vi "CameraServo.vi"(1 "Y":dbl, 2 "X":dbl) -> ()   [LabVIEW 2014]
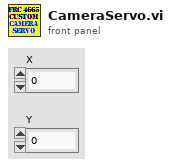
[diagram p1: front panel]
types:
  T1 = typedef "WPI_ServoDeviceRef.ctl" = cluster{"DeviceStatus":errorcluster, "Controller":T2, "PWM Channel":T3, "DeadBand":T4}
  T2 = typedef "FPGA_TypedefDigitalModule.ctl" = enum16{"Controller 1"}
  T3 = typedef "FPGA_DIOPWMChannel.ctl" = enum8{"PWM 0", "PWM 1", "PWM 2", "PWM 3", "PWM 4", "PWM 5", "PWM 6", "PWM 7", "PWM 8", "PWM 9", "PWM MXP 0", "PWM MXP 1", "PWM MXP 2", "PWM MXP 3", "PWM MXP 4", "PWM MXP 5", "PWM MXP 6", "PWM MXP 7", "PWM MXP 8", "PWM MXP 9", "Invalid"}
  T4 = typedef "WPI_PWMDeadband.ctl" = cluster{"Name":string, "maxPositivePwm":i32, "minPositivePwm":i32, "centerPwm":i32, "maxNegativePwm":i32, "minNegativePwm":i32, "angularRange":u16}
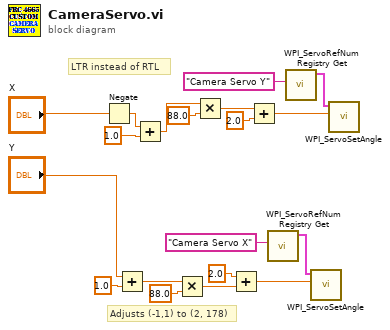
[diagram p0: block diagram]
diagram:
  # "Adjusts (-1,1) to (2, 178)"
  # "LTR instead of RTL"
  n1 = Negate(x="X") -> (-x=w13:dbl)
  n2 = Add(x="Y", y=1.0) -> (x+y=w7:dbl)
  n3 = Add(x=w13, y=1.0) -> (x+y=w12:dbl)
  n4 = Multiply(x=w7, y=88.0) -> (x*y=w5:dbl)
  n5 = Multiply(x=w12, y=88.0) -> (x*y=w15:dbl)
  n6 = Add(x=2.0, y=w5) -> (x+y=w3:dbl)
  n7 = Add(x=w15, y=2.0) -> (x+y=w11:dbl)
  n8 = call <vilib>:"WPI_ServoRefNum Registry Get.vi"("refnum name"="Camera Servo X") -> ("ServoDeviceRef"=w9:T1)  [unwired: 9 in, 1 out]
  n9 = call <vilib>:"WPI_ServoRefNum Registry Get.vi"("refnum name"="Camera Servo Y") -> ("ServoDeviceRef"=w19:T1)  [unwired: 9 in, 1 out]
  n10 = call <vilib>:"WPI_ServoSetAngle.vi"("Angle"=w3, "ServoDeviceRef"=w9) -> ()  [unwired: 8 in, 2 out]
  n11 = call <vilib>:"WPI_ServoSetAngle.vi"("Angle"=w11, "ServoDeviceRef"=w19) -> ()  [unwired: 8 in, 2 out]
